vi "Num Ref Get Value.vi"(8 "error in":errorcluster, 11 "Num Ref":refnum<vi>) -> (0 "error out":errorcluster, 1 "Valid":bool, 2 "Value":variant)   [LabVIEW 2018, in "Main Panel.lvlib" / "Main Panel.lvclass"]
uses:
  Main Panel.lvclass
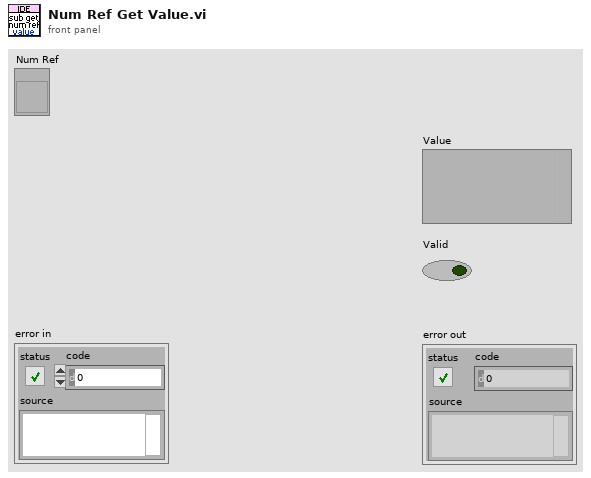
[diagram p1: front panel]
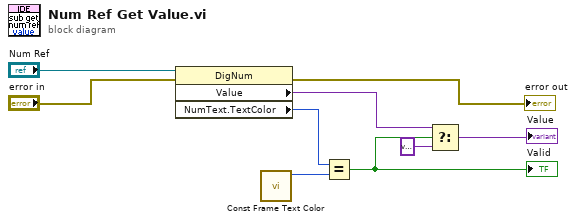
[diagram p0: block diagram]
diagram:
  n1 = property class="DigNum"(reference="Num Ref", error in="error in") -> (error out=→"error out":errorcluster, "Value"=w3:variant, "NumText.TextColor"=w6:u32)  [unwired: 1 out]
  n2 = call "Const Frame Text Color.vi"() -> ("valid num color"=w5:u32)  [unwired: 10 in, 1 out]
  n3 = Equal?(x=w6, y=w5) -> (x = y?=w4:bool)
  "Valid" <- w4
  n4 = Select(t=w3, s=w4, f=variant) -> (s? t:f=→"Value":variant)
